vi "Read from Bank State Decision.vi"(10 "Change?":bool) -> (2 "Next State":T1=enum."Read from Bank")   [LabVIEW 2011]
uses:
  <userlib>/FPGA Library/Code Development/Signal Processing/FFT/Real Sequence from Complex FFT/BRAM State.ctl
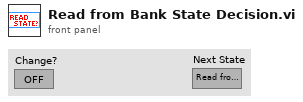
[diagram p1: front panel]
types:
  T1 = typedef "BRAM State.ctl" = enum8{"Write to Bank", "Read from Bank"}
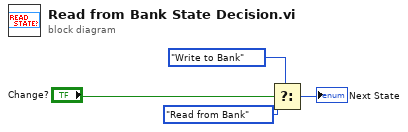
[diagram p0: block diagram]
diagram:
  n1 = Select(t=BRAM_State."Write to Bank", s="Change?", f=BRAM_State."Read from Bank") -> (s? t:f=→"Next State":T1)
